vi "SCPI_Scope_Main.vi"() -> ()   [LabVIEW 2021]
doc: "Recommended Input Signal: 100 kHz, 4 Vpp, sine wave\n\nDevices Supported: Refer to NI Example Finder\n\nThis example configures all the oscilloscope's vertical, horizontal, and triggering properties before every acquisition. It allows you to experiment with numerous configurations, including acquisition types and triggering modes, since it supports nearly the entire functionality of NI-SCOPE. However, it is may be more instructive to consult other examples about specific topics such as FlexRes, Random Interleaved Sampling, and Multi-Record to learn more about these features.\n\nMany parameters are included an the front panel of this example. Notice that the \"min sample rate\" is next to the \"actual sample rate,\" and similarly the \"min record length\" is near the \"actual record length.\" The \"min\" values are specified with the Configure Horizontal Timing VI. NI-SCOPE maintains a constant time per record for each acquisition. So when you specify a min sample rate and a min record length, this determines the amount of time the acquisition should take:\n\n time per record = min record length / min sampling rate. \n\nHowever, oscilloscopes support only a certain number of defined sampling rates, so if the value chosen is not a valid rate, it is rounded to the next higher rate, called the actual sample rate. The actual record length is then calculated in order to maintain the time per record. Both of these values are returned in this example so you can investigate the effects of parameter rounding with your oscilloscope. For more information about parameter coercions, see the NI High Speed Digitizers Help.\n\nThe enforce realtime property allows this example to use Random Interleaved Sampling. See the Random Interleaved Sampling example for more details.\n\nKeep in mind that not all digitizers/oscilloscopes support all the features in this example. The NI High Speed Digitizers Help includes a table of supported features for each device."
uses:
  Controls/Clusts/Scope_Cfg_Clust.ctl
  Controls/Clusts/Resource_Cfg_Clust.ctl
  Controls/Clusts/Vertical_Cfg_Clust.ctl
  Controls/Clusts/Horizontal_Cfg_Clust.ctl
  Controls/Clusts/Trig_Cfg_Clust.ctl
  Controls/Enums/Trig_Type_Enum.ctl
  Controls/Clusts/Trig_Edge_Cfg_Clust.ctl
  Controls/Clusts/Trig_Dig_Cfg_Clust.ctl
  Controls/Enums/Scope_Loop_Enum.ctl
  Controls/Enums/Parser_Loop_Enum.ctl
  Controls/Enums/TCP_Loop_Enum.ctl
  Controls/Enums/HW_Loop_Enum.ctl
  Controls/Clusts/Parse_Loop_Clust.ctl
  Controls/Clusts/Scope_Details.ctl
  <instrlib>/niScope/Utility/niScope Get Channel Name From String.vi
  <instrlib>/niScope/Configure/Trigger/niScope Configure Trigger Immediate.vi
  <instrlib>/niScope/Configure/Trigger/niScope Configure Trigger Edge.vi
  <instrlib>/niScope/Configure/Trigger/niScope Configure Trigger Digital.vi
  <instrlib>/niScope/Acquire/Fetch/niScope Multi Fetch Cluster.vi
panel:
  out "data":string
  out "Index":i32
  in  "Scope":T1={"Resource"={"Resource Name"="Dev1", "Channel Name"="0", "Timeout (s)"=5.0}, "Vert"={"Vertical Range"=5.0, "Vertical Offset"=0.0, "Probe Attenuation"=1.0, "Vertical Coupling"=1}, "Hor"={"Maximum Input Frequency"=0.0, "Min Sample Rate"=10000000.0, "Min Record Length"=1000}, "Trig"={"Trigger Modifier"=2, "Trigger Delay"=0.0, "Reference Position"=50.0, "TrigType"=enum."Immediate", "Edge"={"Coupling"=1, "Trigger Slope"=0, "Trigger Source"="0", "Trigger Level"=0.0}, "Dig"={"Trigger Source"="VAL_PFI_1", "Trigger Slope"=0}}} {"Trig"."Dig"."Trigger Slope" items=["Positive", "Negative"]; "Trig"."Edge"."Trigger Level" format="%.2f"; "Trig"."Edge"."Trigger Slope" items=["Positive", "Negative"]; "Trig"."Edge"."Coupling" items=["AC"=0, "DC"=1, "HF Reject"=3, "LF Reject"=4, "AC Plus HF Reject"=1001]; "Trig"."Reference Position" format="%.1f"; "Trig"."Trigger Delay" format="%#.4p"; "Trig"."Trigger Modifier" items=["None"=1, "Auto Trigger"=2]; "Hor"."Min Sample Rate" step=1000000.0 format="%#.2p"; "Hor"."Maximum Input Frequency" format="%.2f"; "Vert"."Vertical Coupling" items=["AC", "DC", "Ground"]; "Vert"."Probe Attenuation" format="%.1f"; "Vert"."Vertical Offset" format="%.2p"; "Vert"."Vertical Range" format="%.2f"; "Resource"."Timeout (s)" format="%.2f"}
  out "Auto Triggered":bool
  out "Actual Sample Rate":dbl=10000000.0 format="%#.2p"
  out "Actual Record Length":i32=1000
  out "Waveform(s)":T9(graph)
  # "Overview: Demonstrates how to configure vertical, horizontal, and triggering properties and allows you to experiment with numerous configurations, including acquisition types and triggering mode.\nRequirements: NI-SCOPE\nInstructions: \n1. Configure desired acquisition settings.\n2. Run the VI.\n3. Click Stop to stop the VI."
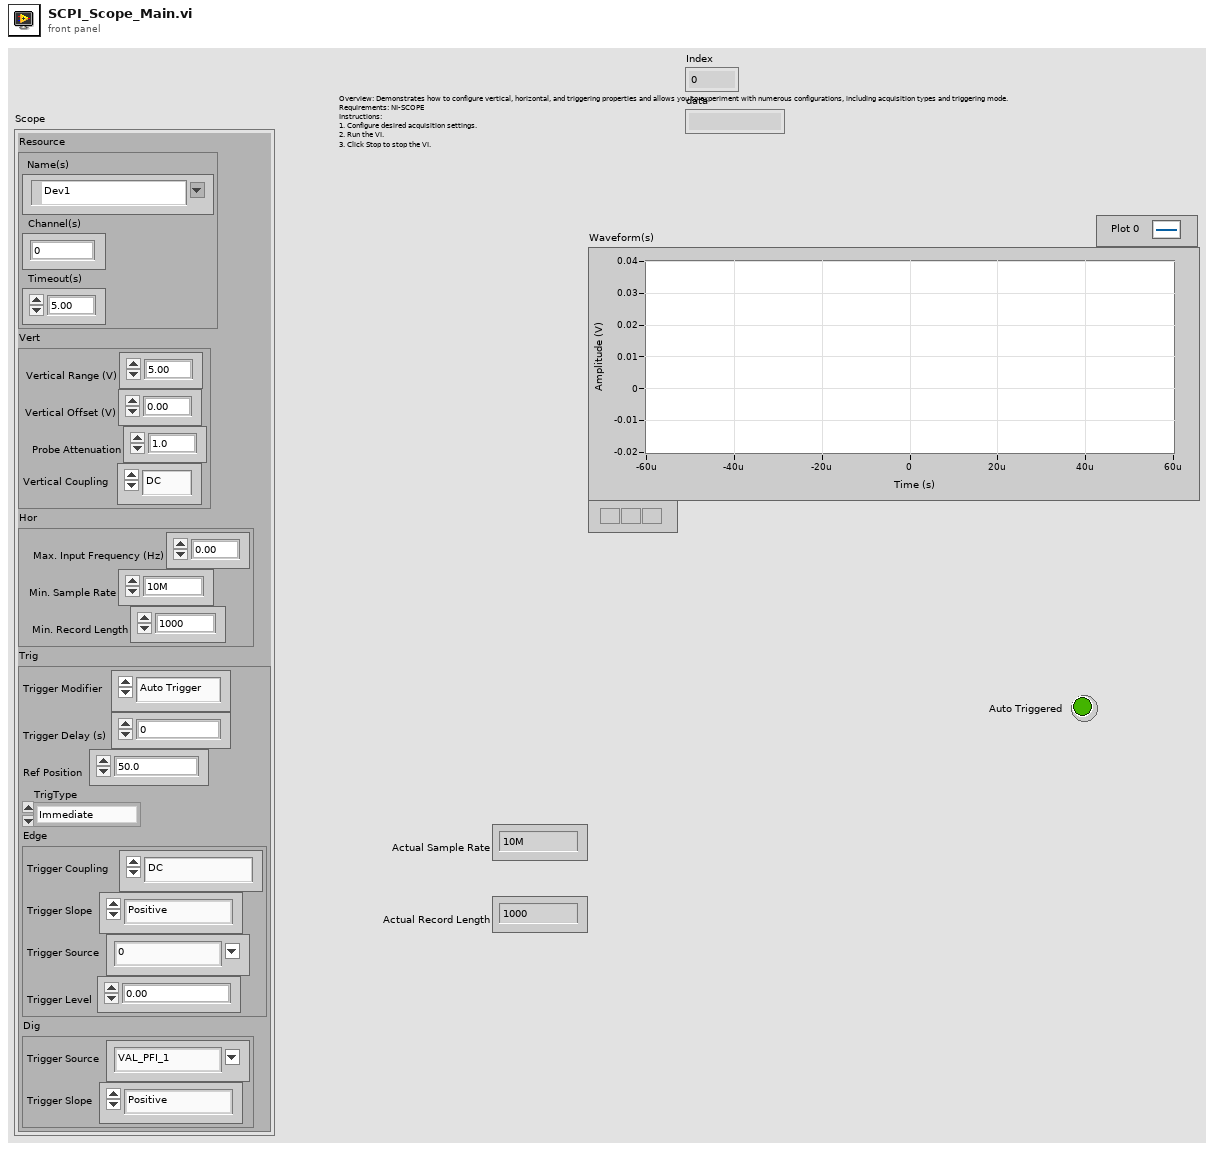
[diagram p1: front panel]
types:
  T1 = typedef "Scope_Cfg_Clust.ctl" = cluster{"Resource":T2, "Vert":T3, "Hor":T4, "Trig":T5}
  T2 = typedef "Resource_Cfg_Clust.ctl" = cluster{"Resource Name":refnum<k15>, "Channel Name":string, "Timeout (s)":dbl}
  T3 = typedef "Vertical_Cfg_Clust.ctl" = cluster{"Vertical Range":dbl, "Vertical Offset":dbl, "Probe Attenuation":dbl, "Vertical Coupling":i32}
  T4 = typedef "Horizontal_Cfg_Clust.ctl" = cluster{"Maximum Input Frequency":dbl, "Min Sample Rate":dbl, "Min Record Length":i32}
  T5 = typedef "Trig_Cfg_Clust.ctl" = cluster{"Trigger Modifier":i32, "Trigger Delay":dbl, "Reference Position":dbl, "TrigType":T6, "Edge":T7, "Dig":T8}
  T6 = typedef "Trig_Type_Enum.ctl" = enum16{"Immediate", "Edge", "Digital"}
  T7 = typedef "Trig_Edge_Cfg_Clust.ctl" = cluster{"Coupling":u16, "Trigger Slope":i32, "Trigger Source":string, "Trigger Level":dbl}
  T8 = typedef "Trig_Dig_Cfg_Clust.ctl" = cluster{"Trigger Source":string, "Trigger Slope":i32}
  T9 = cluster{"relativeInitialX":dbl, "xIncrement":dbl, "wfm":dbl[]}[]
  T10 = typedef "Parse_Loop_Clust.ctl" = cluster{"String_Recvd":string, "String_ToSend":string, "ScopePresent":T11[], "ScopeCfg":T1[]}
  T11 = typedef "Scope_Details.ctl" = cluster{"Alias":string, "Product":string, "SN":string, "Slot":i32, "chans":i32, "State":string}
  T12 = typedef "HW_Loop_Enum.ctl" = cluster{"instrument handle":refnum<k15>, "channel name":string, "TaskRef":refnum<k15>, "Scope":T1}
  T13 = typedef "TCP_Loop_Enum.ctl" = enum16{"TCP_Init", "TCP_Read", "TCP_Write", "TCP_Close"}
  T14 = typedef "Parser_Loop_Enum.ctl" = enum16{"Init", "Receive", "Send", "Parse", "ChkTime", "Close"}
  T15 = typedef "Scope_Loop_Enum.ctl" = enum16{"Init", "Cfg", "Read", "Stop", "Close"}
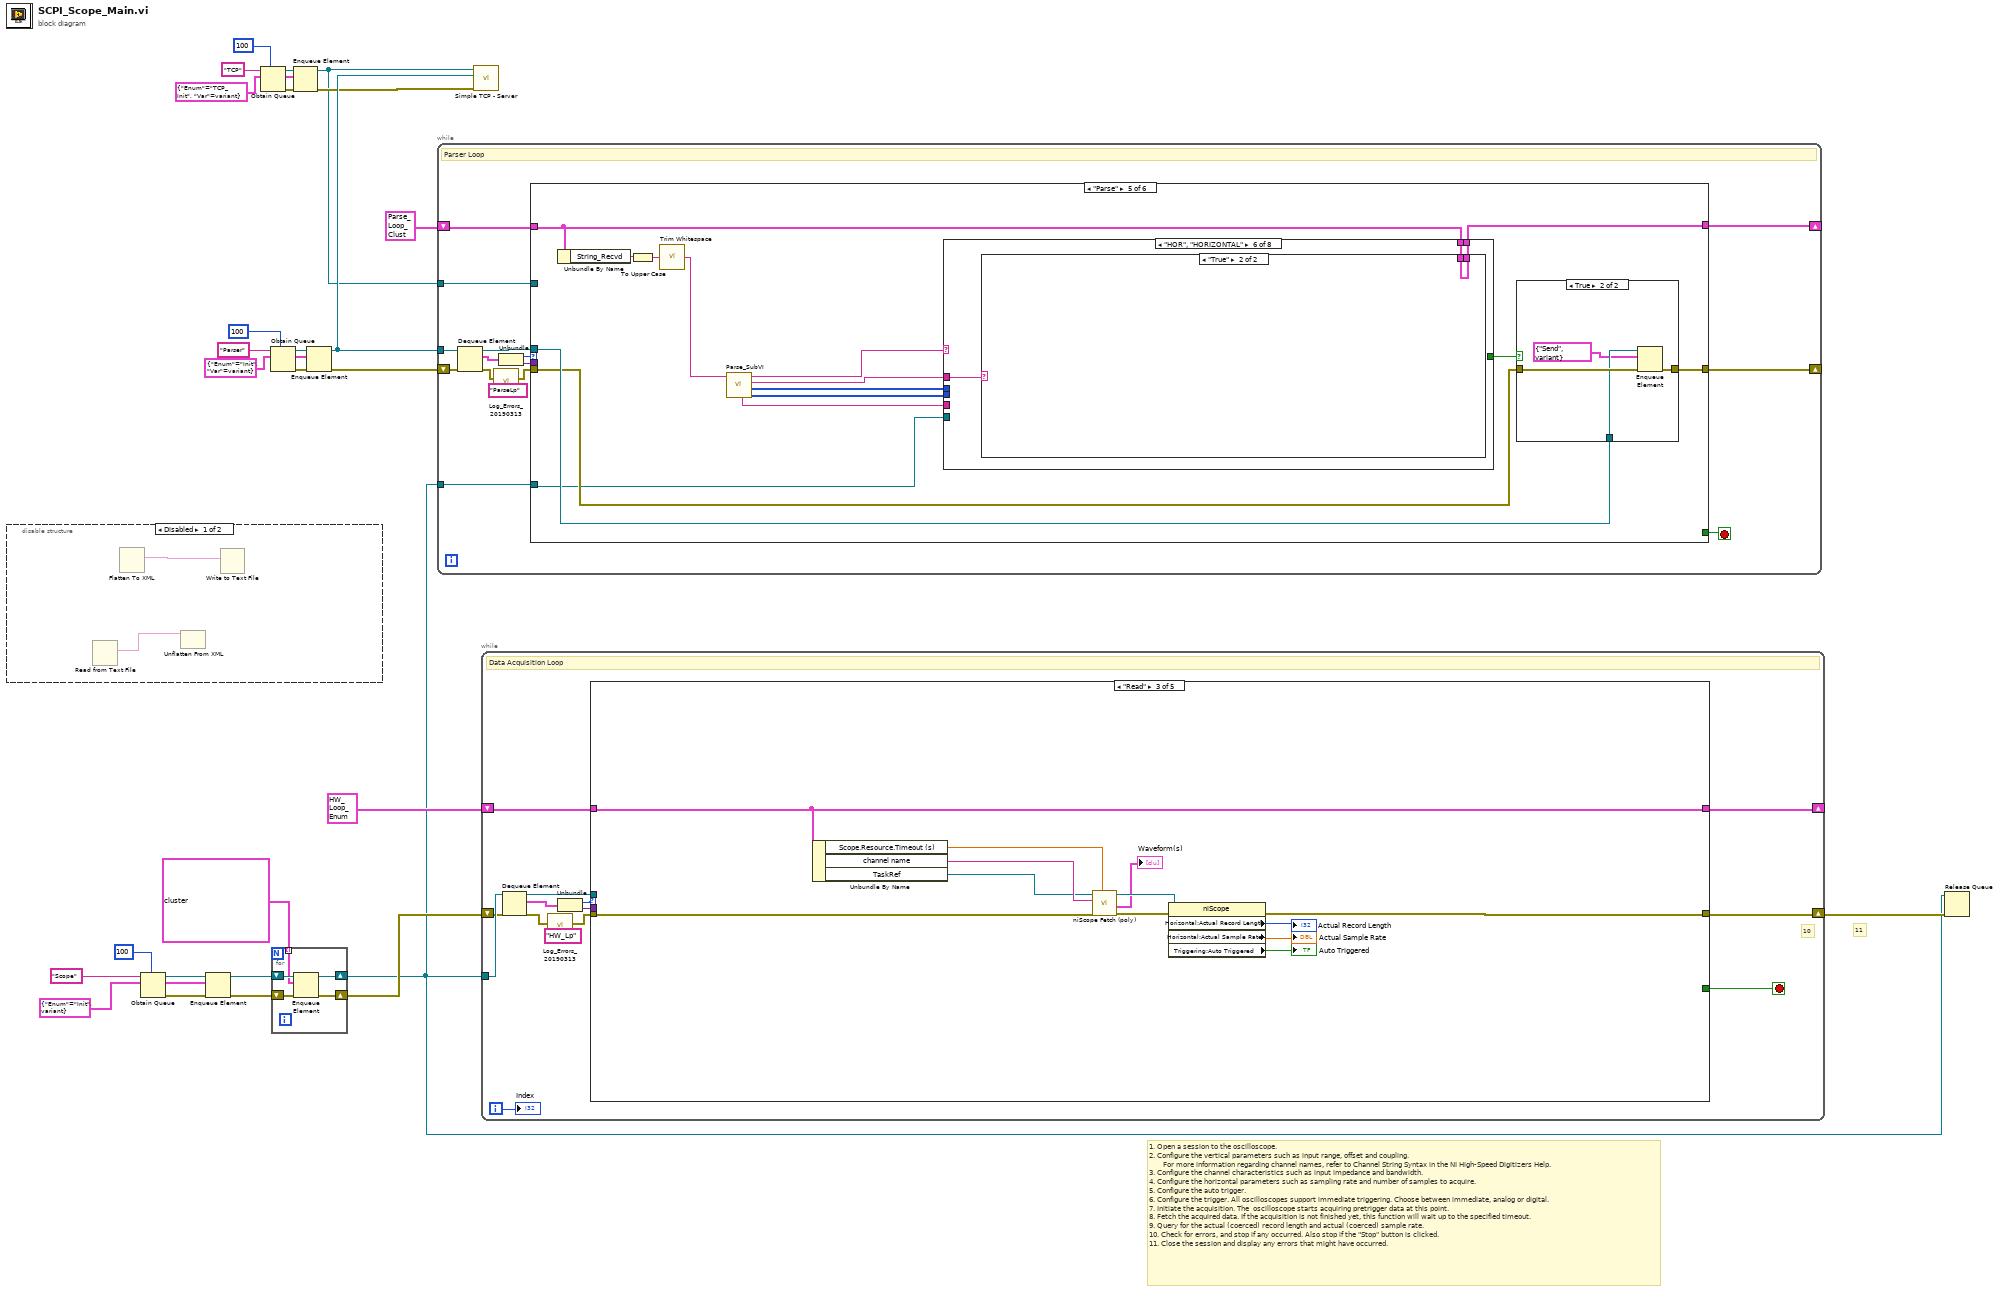
[diagram p0: block diagram]
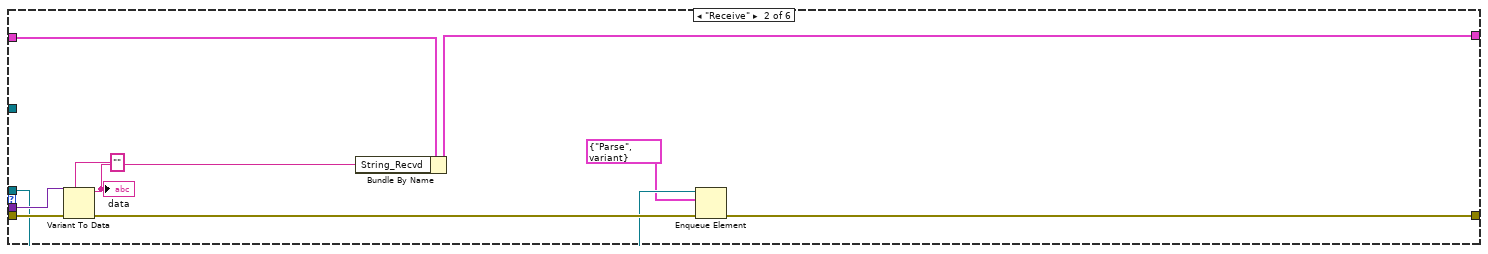
[diagram p4: hidden frame]
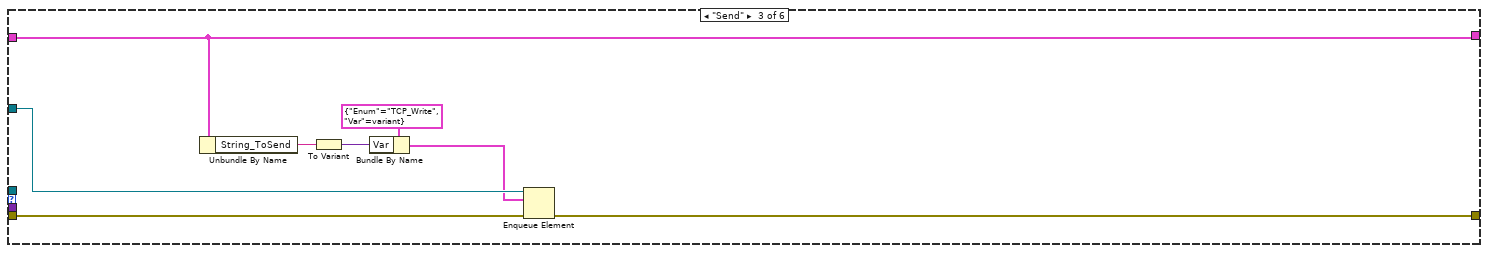
[diagram p5: hidden frame]
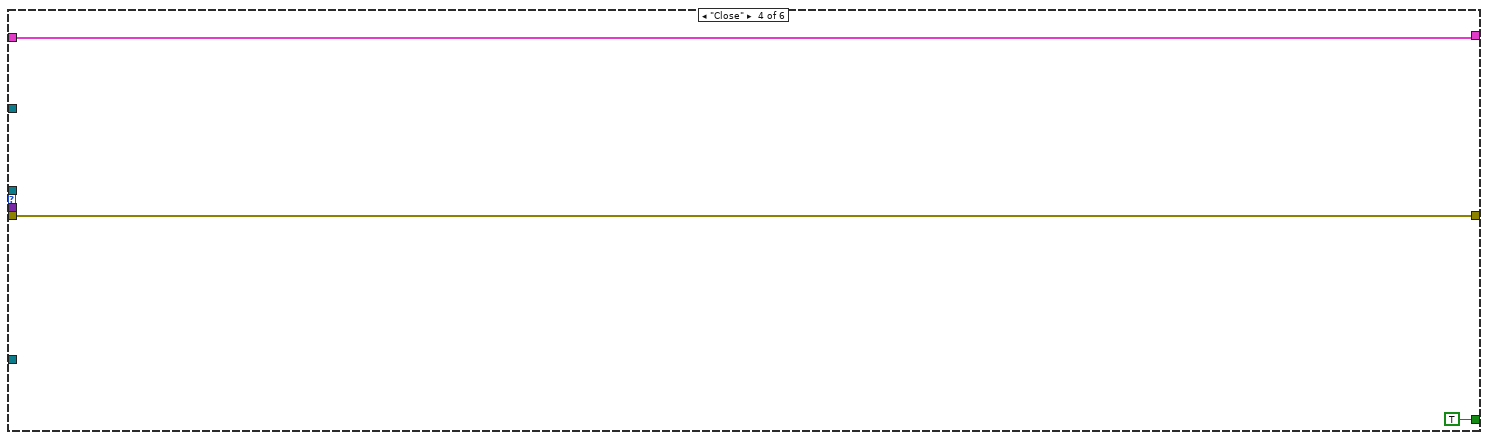
[diagram p6: hidden frame]
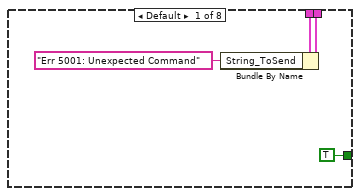
[diagram p7: hidden frame]
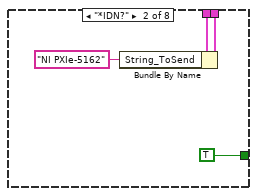
[diagram p8: hidden frame]
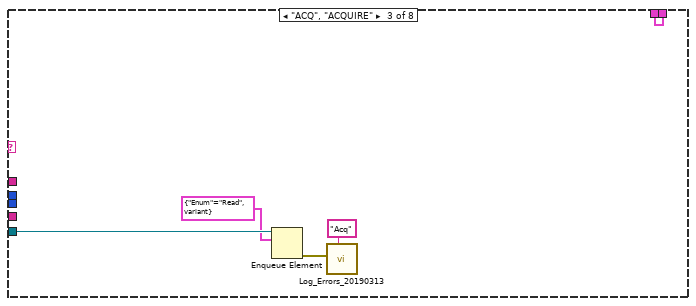
[diagram p9: hidden frame]
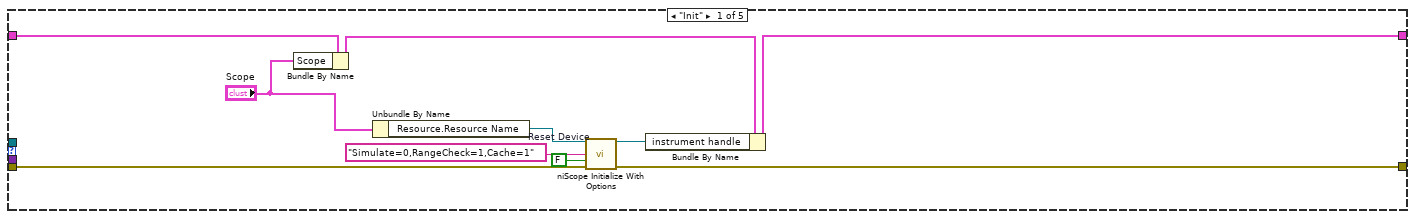
[diagram p17: hidden frame]
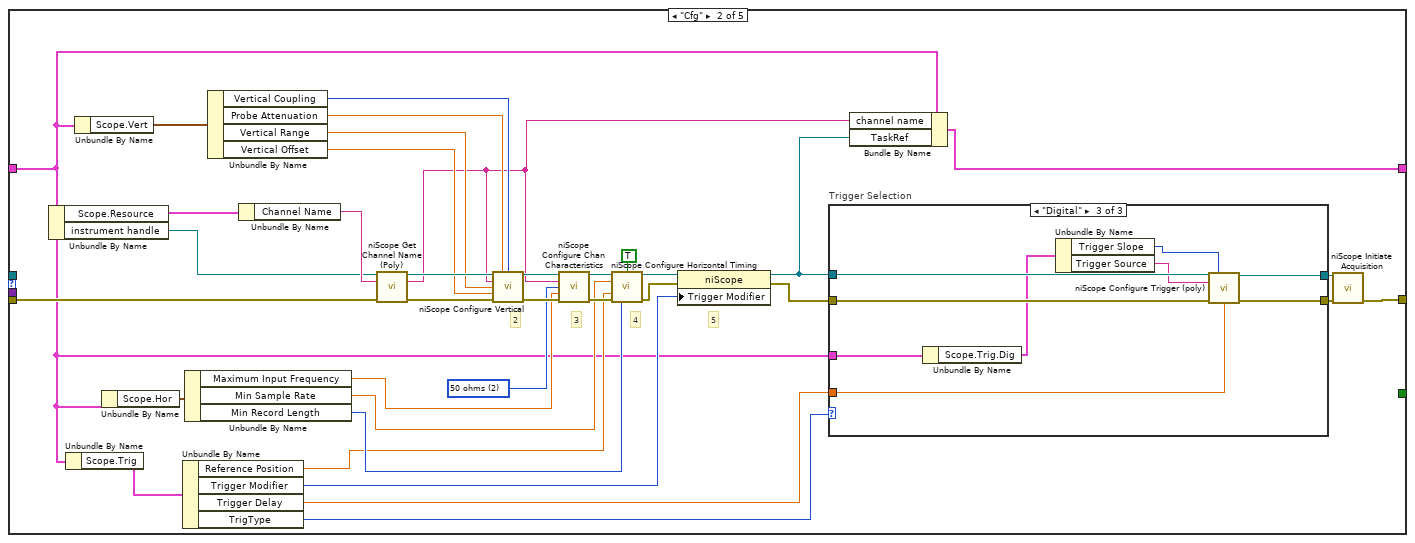
[diagram p18: hidden frame]
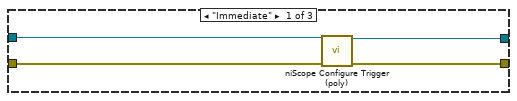
[diagram p19: hidden frame]
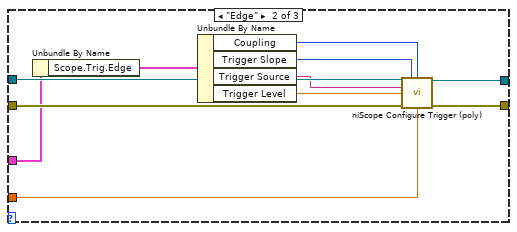
[diagram p20: hidden frame]
diagram:
  w7 = cluster{"Enum":T13, "Var":variant} {"Enum"=enum."TCP_Init", "Var"=variant}
  w14 = cluster{"Enum":T14, "Var":variant} {"Enum"=enum."Init", "Var"=variant}
  w24 = cluster{"Enum":T15, variant} {"Enum"=enum."Init", variant}
  # "1. Open a session to the oscilloscope.\n2. Configure the vertical parameters such as input range, offset and coupling.\n       For more information regarding channel names, refer to Channel String Syntax in the NI High-Speed Digitizers Help.\n3. Configure the channel characteristics such as input impedance and bandwidth.\n4. Configure the horizontal parameters such as sampling rate and number of samples to acquire.\n5. Configure the auto trigger.\n6. Configure the trigger. All oscilloscopes support immediate triggering. Choose between immediate, analog or digital.\n7. Initiate the acquisition. The  oscilloscope starts acquiring pretrigger data at this point.\n8. Fetch the acquired data. If the acquisition is not finished yet, this function will wait up to the specified timeout.\n9. Query for the actual (coerced) record length and actual (coerced) sample rate.\n10. Check for errors, and stop if any occurred. Also stop if the \"Stop\" button is clicked.\n11. Close the session and display any errors that might have occurred."
  # "11"
  n1 = disable-structure shown="Disabled" {
    frame Disabled {
      n2 = Read from Text File() -> (text=w28:string)  [unwired: 4 in, 3 out]
      n3 = Flatten To XML() -> (2:w29:string)  [unwired: 1 in]
      n4 = Unflatten From XML(xml string=w28) -> ()  [unwired: 2 in, 2 out]
      n5 = Write to Text File(text=w29) -> ()  [unwired: 3 in, 3 out]
    }
    frame Enabled {
    }
  }
  n6 = Obtain Queue(max queue size (-1, unlimited)=100, name (unnamed)="Scope", element data type=w24) -> (queue out=w23:refnum<queue>, error out=w25:errorcluster)  [unwired: 2 in, 1 out]
  n7 = Enqueue Element(queue=w23, element=w24, error in (no error)=w25) -> (queue out=w22:refnum<queue>, error out=w21:errorcluster)  [unwired: 1 in, 1 out]
  n8 = Obtain Queue(max queue size (-1, unlimited)=100, name (unnamed)="TCP", element data type=w7) -> (queue out=w6:refnum<queue>, error out=w8:errorcluster)  [unwired: 2 in, 1 out]
  n9 = Obtain Queue(max queue size (-1, unlimited)=100, name (unnamed)="Parser", element data type=w14) -> (queue out=w13:refnum<queue>, error out=w15:errorcluster)  [unwired: 2 in, 1 out]
  n10 = for {
    tunnel: cluster{"Enum":T15, variant}[] [{"Enum"=enum."Cfg", variant}, {"Enum"=enum."Read", variant}, {"Enum"=enum."Stop", variant}, {"Enum"=enum."Close", variant}] -> [w30] mode=indexing
    shift-right: [w34] -> w1
    shift-left: w22 -> [w33]
    shift-right: [w31] -> w20
    shift-left: w21 -> [w32]
    n11 = Enqueue Element(queue=w33, element=w30, error in (no error)=w32) -> (queue out=w34:refnum<queue>, error out=w31:errorcluster)  [unwired: 1 in, 1 out]
  }
  n12 = Enqueue Element(queue=w6, element=w7, error in (no error)=w8) -> (queue out=w2:refnum<queue>, error out=w5:errorcluster)  [unwired: 1 in, 1 out]
  n13 = Enqueue Element(queue=w13, element=w14, error in (no error)=w15) -> (queue out=w11:refnum<queue>, error out=w12:errorcluster)  [unwired: 1 in, 1 out]
  n14 = while {
    shift-right: [w41] -> _
    shift-left: T10 {"String_Recvd"="", "String_ToSend"="", "ScopePresent"=[{"Alias"="PXI1Slot8", "Product"="NI PXIe-5162 (4CH)", "SN"="01B01823", "Slot"=8, "chans"=4, "State"="Unknown"}], "ScopeCfg"=[{"Resource"={"Resource Name"="", "Channel Name"="0", "Timeout (s)"=5.0}, "Vert"={"Vertical Range"=5.0, "Vertical Offset"=0.0, "Probe Attenuation"=1.0, "Vertical Coupling"=1}, "Hor"={"Maximum Input Frequency"=0.0, "Min Sample Rate"=10000000.0, "Min Record Length"=1000}, "Trig"={"Trigger Modifier"=2, "Trigger Delay"=0.0, "Reference Position"=50.0, "TrigType"=enum."Immediate", "Edge"={"Coupling"=1, "Trigger Slope"=0, "Trigger Source"="0", "Trigger Level"=0.0}, "Dig"={"Trigger Source"="VAL_PFI_1", "Trigger Slope"=0}}}]} -> [w42]
    shift-right: [w40] -> _
    shift-left: w12 -> [w37]
    tunnel: w11 -> [w47]
    tunnel: w2 -> [w39]
    tunnel: w1 -> [w38]
    stop <- w43 stop-if-true
    # "Parser Loop"
    n15 = Dequeue Element(queue=w47, error in (no error)=w37) -> (queue out=w45:refnum<queue>, element=w48:cluster{"Enum":T14, "Var":variant})  [unwired: 1 in, 2 out]
    n16 = call "Log_Errors_20190313.vi"("LoopName"="ParseLp", "error in"=w37) -> ("error out"=w36:errorcluster)  [unwired: 9 in]
    n17 = Unbundle(w48) -> ("Enum"=w46:T14, "Var"=w44:variant)
    n18 = case shown="\"Parse\"" w46 {
      tunnel: w45 -> [_ w52 _ _ w84 _]
      tunnel: w36 -> [w50 w60 w66 w69 w80 w113]
      tunnel: w44 -> [_ w58 _ _ _ _]
      tunnel: [_ _ _ TRUE _ _] -> w43
      tunnel: w42 -> [w49 w57 w68 w70 w83 w114]
      tunnel: [w49 w55 w68 w70 w82 w114] -> w41
      tunnel: [w50 w53 w67 w69 w85 w113] -> w40
      tunnel: w39 -> [_ _ w65 _ _ _]
      tunnel: w38 -> [_ _ _ _ w72 _]
      frame "Init" {
      }
      frame "Receive" {
        n19 = Variant To Data(error in=w60, type="", Variant=w58) -> (data=w56:string, error out=w54:errorcluster)
        "data" <- w56
        n20 = Bundle By Name(cluster=w57, "String_Recvd"=w56) -> (w55:T10)
        n21 = Enqueue Element(queue=w52, element=cluster{T14, variant} {enum."Parse", variant}, error in (no error)=w54) -> (error out=w53:errorcluster)  [unwired: 1 in, 2 out]
      }
      frame "Send" {
        n22 = Unbundle By Name(w68) -> ("String_ToSend"=w63:string)
        n23 = To Variant(anything=w63) -> (Variant=w61:variant)
        n24 = Bundle By Name(cluster=cluster{"Enum":T13, "Var":variant} {"Enum"=enum."TCP_Write", "Var"=variant}, "Var"=w61) -> (w64:cluster{"Enum":T13, "Var":variant})
        n25 = Enqueue Element(queue=w65, element=w64, error in (no error)=w66) -> (error out=w67:errorcluster)  [unwired: 1 in, 2 out]
      }
      frame "Close" {
      }
      frame "Parse" {
        n26 = Unbundle By Name(w83) -> ("String_Recvd"=w86:string)
        n27 = To Upper Case(1:w86) -> (0:w79:string)
        n28 = call <vilib>:"Trim Whitespace.vi"("string"=w79) -> ("trimmed string"=w78:string)  [unwired: 1 in]
        n29 = call "Parse_SubVI.vi"("SCPI String"=w78) -> ("Channel_Array"=w74:i32[], "Device_Array"=w75:i32[], "SubCommand"=w76:string, "Command"=w77:string, "Parameters"=w73:string)  [unwired: 6 in]
        n30 = case shown="\"HOR\", \"HORIZONTAL\"" w77 {
          tunnel: w83 -> [w88 w94 w99 w100 w101 w103 w106 w107]
          tunnel: [w87 w93 w99 w100 w101 w104 w106 w107] -> w82
          tunnel: [TRUE TRUE _ _ _ _ _ _] -> w81
          tunnel: w76 -> [_ _ _ _ _ w102 _ _]
          tunnel: w75 -> [_ _ _ _ _ _ _ _]
          tunnel: w74 -> [_ _ _ _ _ _ _ _]
          tunnel: w73 -> [_ _ _ _ _ _ _ _]
          tunnel: w72 -> [_ _ w98 _ _ _ _ _]
          frame Default {
            n31 = Bundle By Name(cluster=w88, "String_ToSend"="Err 5001: Unexpected Command") -> (w87:T10)
          }
          frame "*IDN?" {
            n32 = Bundle By Name(cluster=w94, "String_ToSend"="NI PXIe-5162") -> (w93:T10)
          }
          frame "ACQ", "ACQUIRE" {
            n33 = Enqueue Element(queue=w98, element=cluster{"Enum":T15, variant} {"Enum"=enum."Read", variant}) -> (error out=w96:errorcluster)  [unwired: 2 in, 2 out]
            n34 = call "Log_Errors_20190313.vi"("LoopName"="Acq", "error in"=w96) -> ()  [unwired: 9 in, 1 out]
          }
          frame "CH", "CHANNEL" {
          }
          frame "DAT", "DATA" {
          }
          frame "HOR", "HORIZONTAL" {
            n35 = case shown="\"True\"" w102 {
              tunnel: [_ w105] -> w104
              tunnel: w103 -> [_ w105]
              frame "False", Default {
              }
              frame "True" {
              }
            }
          }
          frame "TRIG", "TRIGGER" {
          }
          frame "VERT", "VERTICAL" {
          }
        }
        n36 = case shown="True" w81 {
          tunnel: w80 -> [w108 w112]
          tunnel: [w108 w111] -> w85
          tunnel: w84 -> [_ w110]
          frame False {
          }
          frame True {
            n37 = Enqueue Element(queue=w110, element=cluster{T14, variant} {enum."Send", variant}, error in (no error)=w112) -> (error out=w111:errorcluster)  [unwired: 1 in, 2 out]
          }
        }
      }
      frame "ChkTime" {
      }
    }
  }
  n38 = call "Simple TCP - Server.vi"("error"=w5, "ParserQueue"=w11, "TCP_Queue"=w2) -> ()  [unwired: 9 in]
  n39 = while {
    shift-right: [w121] -> w18
    shift-left: w20 -> [w117]
    shift-right: [w120] -> _
    shift-left: T12 {"instrument handle"="", "channel name"="", "TaskRef"="", "Scope"={"Resource"={"Resource Name"="5162", "Channel Name"="0", "Timeout (s)"=5.0}, "Vert"={"Vertical Range"=5.0, "Vertical Offset"=0.0, "Probe Attenuation"=1.0, "Vertical Coupling"=1}, "Hor"={"Maximum Input Frequency"=0.0, "Min Sample Rate"=10000000.0, "Min Record Length"=1000}, "Trig"={"Trigger Modifier"=2, "Trigger Delay"=0.0, "Reference Position"=50.0, "TrigType"=enum."Immediate", "Edge"={"Coupling"=1, "Trigger Slope"=0, "Trigger Source"="0", "Trigger Level"=0.0}, "Dig"={"Trigger Source"="VAL_PFI_1", "Trigger Slope"=0}}}} ("HW") -> [w127]
    tunnel: w1 -> [w126]
    i -> [w118]
    stop <- w119 stop-if-true
    # "10"
    # "Data Acquisition Loop"
    n40 = Dequeue Element(queue=w126, error in (no error)=w117) -> (queue out=w125:refnum<queue>, element=w124:cluster{"Enum":T15, variant})  [unwired: 1 in, 2 out]
    n41 = call "Log_Errors_20190313.vi"("LoopName"="HW_Lp", "error in"=w117) -> ("error out"=w116:errorcluster)  [unwired: 9 in]
    n42 = Unbundle(w124) -> ("Enum"=w123:T15, w122:variant)
    n43 = case shown="\"Read\"" w123 {
      tunnel: [w132 w167 w198 w212 w215] -> w121
      tunnel: w116 -> [w133 w159 w199 w213 w215]
      tunnel: w127 -> [w130 w141 w201 w210 w214]
      tunnel: w125 -> [_ _ _ _ _]
      tunnel: w122 -> [_ _ _ _ _]
      tunnel: [w131 w140 w201 w210 w214] -> w120
      tunnel: [_ _ _ _ TRUE ("Stop")] -> w119
      frame "Init" {
        w134 = FALSE  # Reset Device
        n44 = Bundle By Name(cluster=w130, "Scope"="Scope") -> (w129:T12)
        n45 = Unbundle By Name("Scope") -> ("Resource.Resource Name"=w136:refnum<k15>)
        n46 = call <instrlib>:"niScope Initialize With Options.vi"("resource name"=w136, "option string"="Simulate=0,RangeCheck=1,Cache=1", "reset device"=w134, "error in"=w133) -> ("instrument handle"=w137:refnum<k15>, "error out"=w132:errorcluster)  [unwired: 10 in]
        n47 = Bundle By Name(cluster=w129, "instrument handle"=w137) -> (w131:T12)
      }
      frame "Cfg" {
        w169 = u32 2 items=["1 mega ohm"=0, "50 ohms"=2] ("Input Impedance")
        # "5"
        # "2"
        # "3"
        # "4"
        n48 = Unbundle By Name(w141) -> ("Scope.Resource"=w145:T2, "instrument handle"=w142:refnum<k15>)
        n49 = Unbundle By Name(w141) -> ("Scope.Trig"=w144:T5)
        n50 = Unbundle By Name(w141) -> ("Scope.Vert"=w146:T3)
        n51 = Unbundle By Name(w141) -> ("Scope.Hor"=w143:T4)
        n52 = Unbundle By Name(w144) -> ("Reference Position"=w150:dbl, "Trigger Modifier"=w149:i32, "Trigger Delay"=w148:dbl, "TrigType"=w147:T6)
        n53 = Unbundle By Name(w143) -> ("Maximum Input Frequency"=w153:dbl, "Min Sample Rate"=w152:dbl, "Min Record Length"=w151:i32)
        n54 = Unbundle By Name(w146) -> ("Vertical Coupling"=w157:i32, "Probe Attenuation"=w156:dbl, "Vertical Range"=w155:dbl, "Vertical Offset"=w154:dbl)
        n55 = Unbundle By Name(w145) -> ("Channel Name"=w158:string)
        n56 = call-poly <instrlib>:"niScope Get Channel Name (Poly).vi"("instrument handle"=w142, "index"=w158, "error in"=w159) -> ("instrument handle out"=w161:refnum<k15>, "channel name"=w139:string, "error out"=w160:errorcluster)  [unwired: 10 in]
        n57 = call <instrlib>:"niScope Configure Vertical.vi"("instrument handle"=w161, "probe attenuation"=w156, "vertical coupling"=w157, "channels"=w139, "vertical range"=w155, "vertical offset"=w154, "error in"=w160) -> ("instrument handle out"=w173:refnum<k15>, "error out"=w172:errorcluster)  [unwired: 7 in]
        n58 = call <instrlib>:"niScope Configure Chan Characteristics.vi"("instrument handle"=w173, "channels"=w139, "input impedance"=w169, "maximum input frequency"=w153, "error in"=w172) -> ("instrument handle out"=w170:refnum<k15>, "error out"=w171:errorcluster)  [unwired: 9 in]
        n59 = call <instrlib>:"niScope Configure Horizontal Timing.vi"("instrument handle"=w170, "enforce realtime"=TRUE ("Enforce Realtime"), "min sample rate"=w152, "reference position"=w150, "error in"=w171, "min record length"=w151) -> ("instrument handle out"=w165:refnum<k15>, "error out"=w164:errorcluster)  [unwired: 8 in]
        n60 = property on="Property Node" class="niScope"(reference=w165, error in=w164, "Trigger Modifier"=w149) -> (reference out=w138:refnum<k15>, error out=w163:errorcluster)
        n61 = case "Trigger Selection" shown="\"Digital\"" w147 {
          tunnel: w163 -> [w177 w188 w197]
          tunnel: [w174 w184 w193] -> w166
          tunnel: w138 -> [w176 w187 w196]
          tunnel: [w175 w185 w194] -> w168
          tunnel: w148 -> [_ w186 w195]
          tunnel: w141 -> [_ w178 w190]
          frame "Immediate" {
            n62 = call-poly <instrlib>:"niScope Configure Trigger (poly).vi"("instrument handle"=w176, "error in"=w177) -> ("instrument handle out"=w175:refnum<k15>, "error out"=w174:errorcluster)  [unwired: 12 in]
          }
          frame "Edge" {
            n63 = Unbundle By Name(w178) -> ("Scope.Trig.Edge"=w179:T7)
            n64 = Unbundle By Name(w179) -> ("Coupling"=w183:u16, "Trigger Slope"=w182:i32, "Trigger Source"=w181:string, "Trigger Level"=w180:dbl)
            n65 = call-poly <instrlib>:"niScope Configure Trigger (poly).vi"("instrument handle"=w187, "trigger slope"=w182, "trigger coupling"=w183, "trigger source"=w181, "trigger level"=w180, "error in"=w188, "trigger delay"=w186) -> ("instrument handle out"=w185:refnum<k15>, "error out"=w184:errorcluster)  [unwired: 7 in]
          }
          frame "Digital" {
            n66 = Unbundle By Name(w190) -> ("Scope.Trig.Dig"=w189:T8)
            n67 = Unbundle By Name(w189) -> ("Trigger Slope"=w191:i32, "Trigger Source"=w192:string)
            n68 = call-poly <instrlib>:"niScope Configure Trigger (poly).vi"("instrument handle"=w196, "trigger slope"=w191, "trigger source"=w192, "error in"=w197, "trigger delay"=w195) -> ("instrument handle out"=w194:refnum<k15>, "error out"=w193:errorcluster)  [unwired: 9 in]
          }
        }
        n69 = Bundle By Name(cluster=w141, "channel name"=w139, "TaskRef"=w138) -> (w140:T12)
        n70 = call <instrlib>:"niScope Initiate Acquisition.vi"("instrument handle"=w168, "error in"=w166) -> ("error out"=w167:errorcluster)  [unwired: 12 in, 1 out]
      }
      frame "Read" {
        n71 = Unbundle By Name(w201) -> ("Scope.Resource.Timeout (s)"=w208:dbl, "channel name"=w209:string, "TaskRef"=w200:refnum<k15>)
        n72 = call-poly <instrlib>:"niScope Fetch (poly).vi"("timeout"=w208, "error in"=w199, "channels"=w209, "instrument handle"=w200) -> ("error out"=w204:errorcluster, "waveform"=→"Waveform(s)":T9, "instrument handle out"=w203:refnum<k15>)  [unwired: 4 in, 1 out]
        n73 = property class="niScope"(reference=w203, error in=w204) -> (error out=w198:errorcluster, "Horizontal:Actual Record Length"=→"Actual Record Length":i32, "Horizontal:Actual Sample Rate"=→"Actual Sample Rate":dbl, "Triggering:Auto Triggered"=→"Auto Triggered":bool)  [unwired: 1 out]
      }
      frame "Stop" {
        # "Close task to release device"
        n74 = Unbundle By Name(w210) -> ("TaskRef"=w211:refnum<k15>)
        n75 = call <instrlib>:"niScope Close.vi"("instrument handle"=w211, "error in"=w213) -> ("error out"=w212:errorcluster)  [unwired: 13 in]
      }
      frame "Close" {
      }
    }
    "Index" <- w118
  }
  n76 = Release Queue(queue=w1, error in (no error)=w18) -> ()  [unwired: 1 in, 3 out]
